vi "Gigatronics910_SetFreqLevel.vi"(0 "GPIB Address":string="5", 1 "Frequency (GHz)":dbl=6.0 format="%#_9g", 2 "Power (dBm)":dbl=-70.0) -> ()   [LabVIEW 2014]
panel:
  # "2nd tone GPIB = 5\n1st tone GPIB = 6"
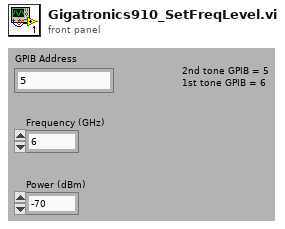
[diagram p1: front panel]
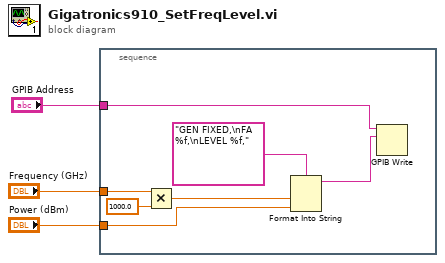
[diagram p0: block diagram]
diagram:
  n1 = stacked-sequence {
    tunnel: "GPIB Address" -> [w10]
    tunnel: "Frequency (GHz)" -> [w7]
    tunnel: "Power (dBm)" -> [w4]
    frame #0 {
      n2 = Multiply(x=w7, y=1000.0) -> (x*y=w6:dbl)
      n3 = Format Into String(format string="GEN FIXED,\nFA %f,\nLEVEL %f,", w6, w4) -> (resulting string=w8:string)  [unwired: 2 in, 1 out]
      n4 = GPIB Write(0:w10, 1:w8) -> ()  [unwired: 2 in, 3 out]
    }
  }
